vi "Ring management test.vi"() -> ()   [LabVIEW 2016]
uses:
  <vilib>/Utility/miscctls.llb/LVStringsAndValuesArrayTypeDef_U16.ctl
panel:
  in  "stop":bool
  in  "Selection":enum16{"Tektronix", "PicoScope"}(ring)
  in  "Parameters":u16(ring) items=["0.5", "1", "5"]
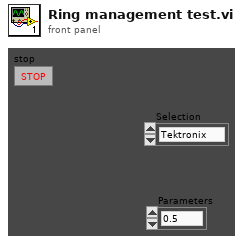
[diagram p1: front panel]
types:
  T1 = typedef "LVStringsAndValuesArrayTypeDef_U16.ctl" = cluster{"String":string, "Value":u16}[]
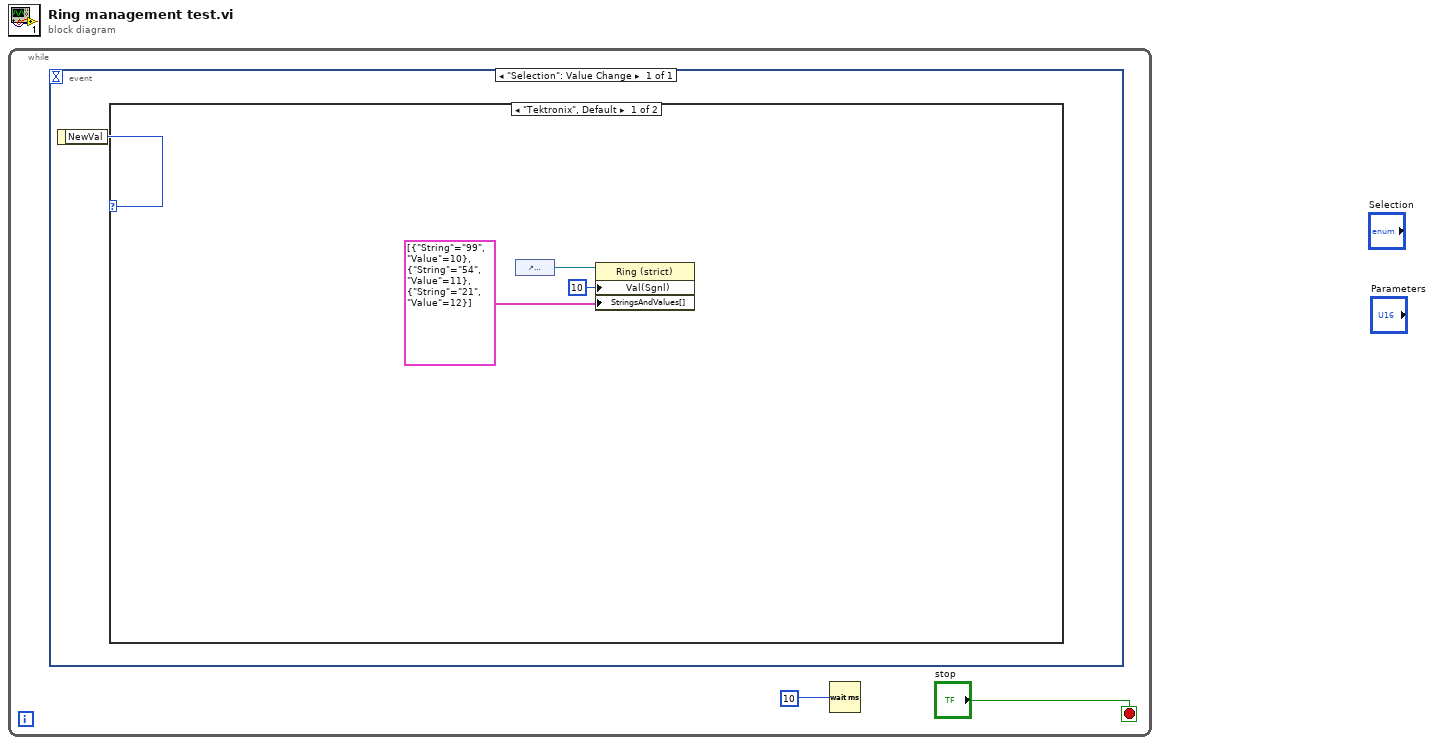
[diagram p0: block diagram]
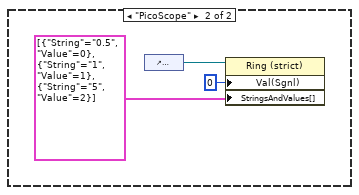
[diagram p2: hidden frame]
diagram:
  n1 = while {
    stop <- "stop" stop-if-true
    n2 = event shown="[0] \"Selection\": Value Change" {
      selector: _ -> [_]
      dyn-events: _ -> [_]
      timeout: _ -> [_]
      event "Selection": Value Change {
        n3 = event-data() -> ("NewVal"=w3:enum16{"Tektronix", "PicoScope"})  [unwired: 1 in]
        n4 = case shown="\"Tektronix\", Default" w3 {
          frame "Tektronix", Default {
            n5 = control-ref of="Parameters"() -> (w4:refnum<vi>)
            n6 = property class="Ring (strict)"(reference=w4, "Val(Sgnl)"=u16 10 ("Value (Signaling)"), "StringsAndValues[]"=T1 [{"String"="99", "Value"=10}, {"String"="54", "Value"=11}, {"String"="21", "Value"=12}] ("Strings And Values []")) -> ()  [unwired: 1 in, 2 out]
          }
          frame "PicoScope" {
            n7 = control-ref of="Parameters"() -> (w9:refnum<vi>)
            n8 = property class="Ring (strict)"(reference=w9, "Val(Sgnl)"=u16 0 ("Value (Signaling)"), "StringsAndValues[]"=T1 [{"String"="0.5", "Value"=0}, {"String"="1", "Value"=1}, {"String"="5", "Value"=2}] ("Strings And Values []")) -> ()  [unwired: 1 in, 2 out]
          }
        }
      }
    }
    n9 = Wait (ms)(milliseconds to wait=u32 10 ("millisecond timer value")) -> ()  [unwired: 1 out]
  }
